vi "Mixed mode s-parameter conversion.vi"() -> ()   [LabVIEW 2020]
uses:
  <vilib>/Analysis/baseanly.llb/Complex A x B.vi
  <vilib>/addons/HF Network Analysis/Support VIs/Read SnP File (SnP).vi
  <vilib>/Analysis/Matrix/Numeric/Conversions/Array To Matrix - CA2.vi
  <vilib>/Analysis/Matrix/Numeric/Multiply/Multiply - CM,C.vi
  <vilib>/Analysis/baseanly.llb/Complex Inverse Matrix.vi
  <vilib>/Analysis/Matrix/Numeric/Conversions/Matrix To Array - CM.vi
  <vilib>/addons/HF Network Analysis/NI_HFNetworkAnalysis.lvlib
  <vilib>/Analysis/Matrix/NI_Matrix.lvlib
  <vilib>/Analysis/NI_AALBase.lvlib
panel:
  in  "Mixed mode port assignment":enum16{"a", "b"}(ring)
  in  "Direction":T1(ring)
  in  "SnP File Path":path
  # "Input file"
  # "Port assignment a (Keysight, R&S)\nSdd11 Sdc11 Sdd12 Sdc12\nScd11 Scc11  Scd12 Scc12\nSdd21 Sdc21 Sdd22 Sdc22\nScd21 Scc21 Scd22 Scc22\n\nPort assignment b (Dr. Bogatin, Dr. Dunsmore, ADS example)\nSdd11 Sdd12 Sdc11 Sdc12\nSdd21 Sdd22  Sdc21 Sdc22\nScd11 Scd12 Scc11 Scc12\nScd21 Scd22 Scc21 Scc22"
  # "Port assignment 4-port common mode\nS11 S12 S13 S14\nS21 S22 S23 S24\nS31 S32 S33 S34\nS41 S42 S43 S44"
  # "Single ended\nports"
  # "1\n\n3"
  # "2\n\n4"
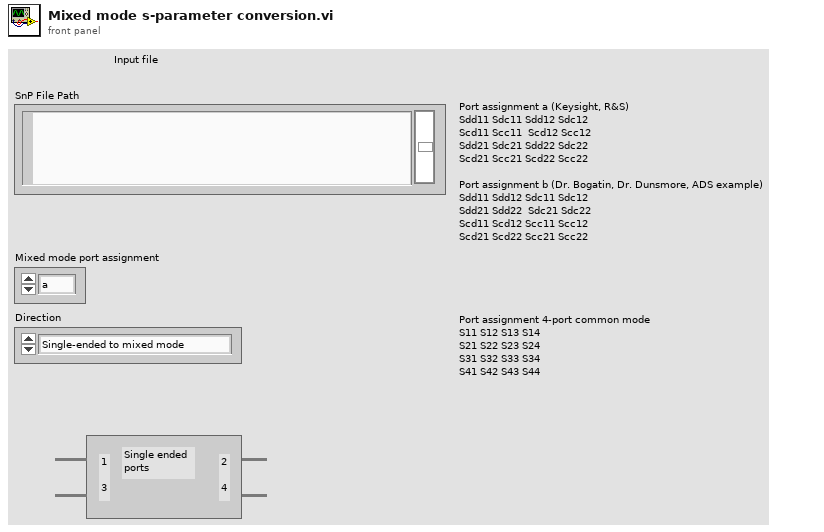
[diagram p1: front panel]
types:
  T1 = enum16{"Single-ended to mixed mode", "Mixed mode to single-ended"}
  T2 = typedef "NI_Matrix.lvlib/ComplexMatrix.ctl" = cdb[][]
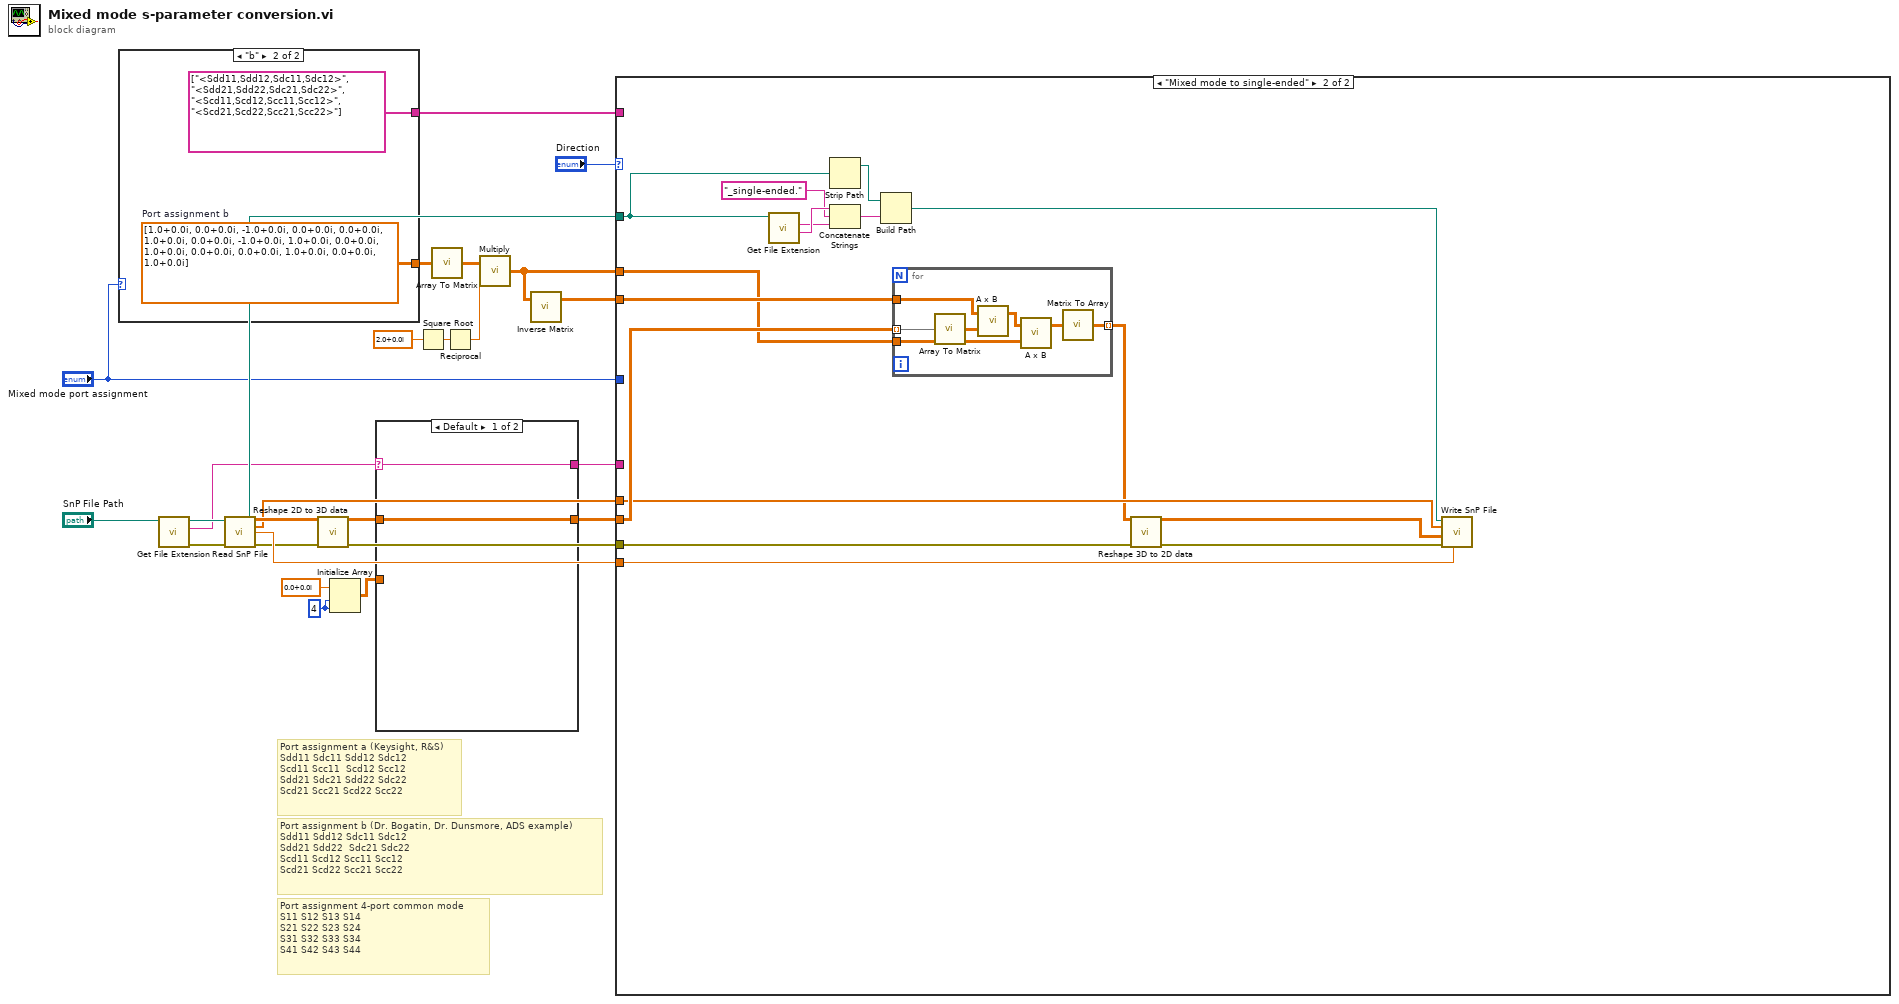
[diagram p0: block diagram]
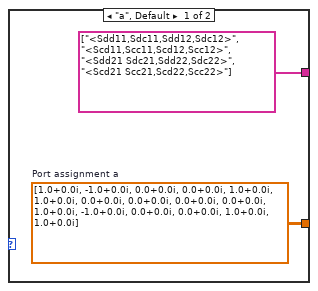
[diagram p2: hidden frame]
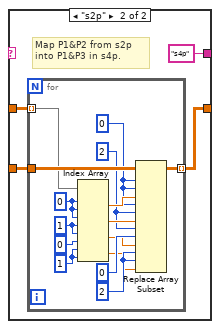
[diagram p3: hidden frame]
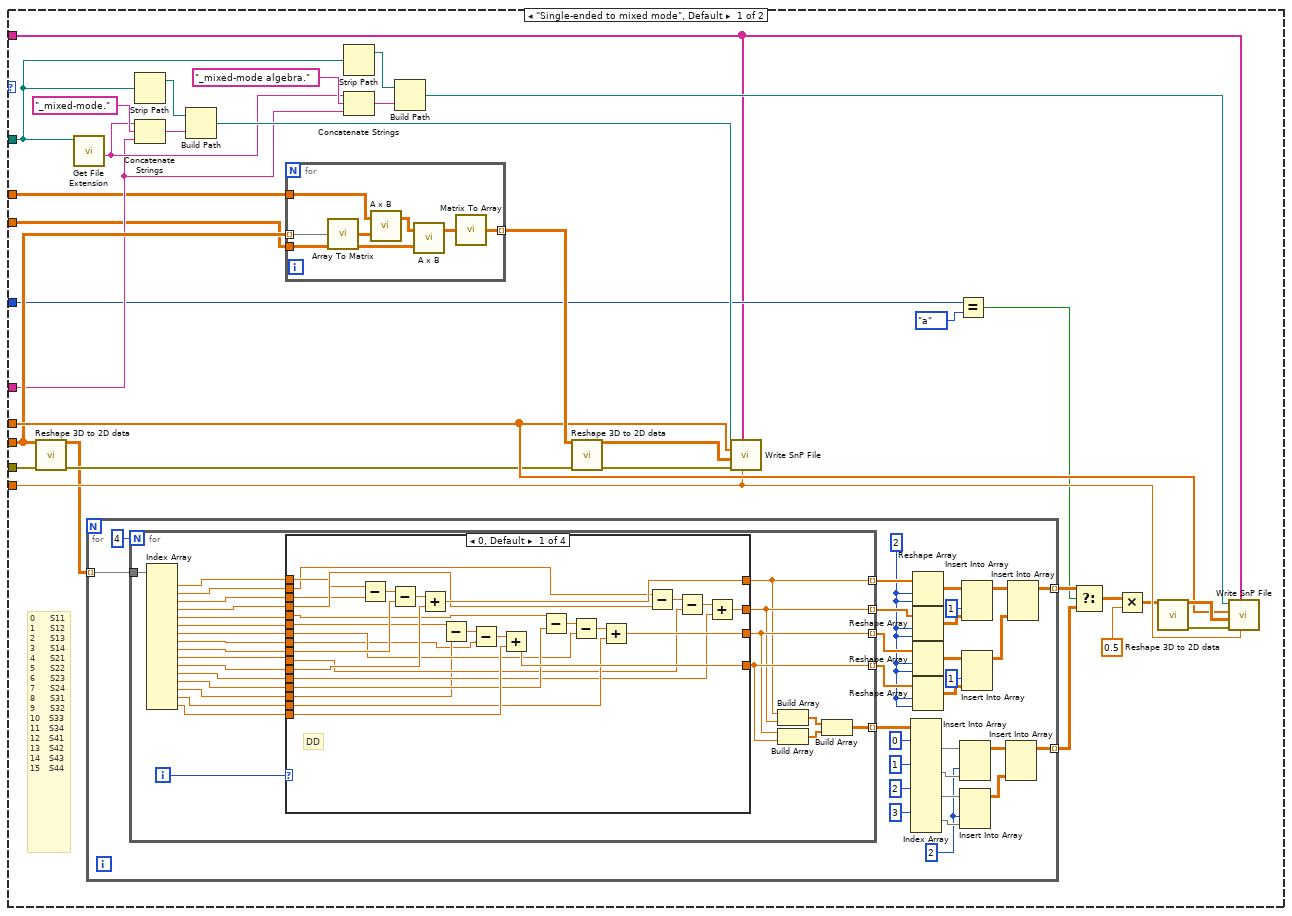
[diagram p4: hidden frame]
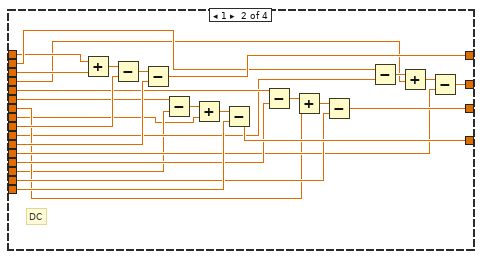
[diagram p5: hidden frame]
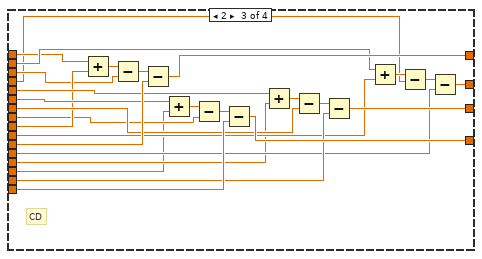
[diagram p6: hidden frame]
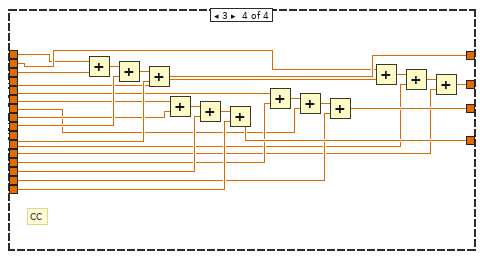
[diagram p7: hidden frame]
diagram:
  w3 = 4 ("dimension size")
  # "Port assignment 4-port common mode\nS11 S12 S13 S14\nS21 S22 S23 S24\nS31 S32 S33 S34\nS41 S42 S43 S44"
  # "Port assignment b (Dr. Bogatin, Dr. Dunsmore, ADS example)\nSdd11 Sdd12 Sdc11 Sdc12\nSdd21 Sdd22  Sdc21 Sdc22\nScd11 Scd12 Scc11 Scc12\nScd21 Scd22 Scc21 Scc22"
  # "Port assignment a (Keysight, R&S)\nSdd11 Sdc11 Sdd12 Sdc12\nScd11 Scc11  Scd12 Scc12\nSdd21 Sdc21 Sdd22 Sdc22\nScd21 Scc21 Scd22 Scc22"
  n1 = case shown="\"b\"" "Mixed mode port assignment" {
    tunnel: [w27 w29] -> w6
    tunnel: [string[] ["<Sdd11,Sdc11,Sdd12,Sdc12>", "<Scd11,Scc11,Scd12,Scc12>", "<Sdd21 Sdc21,Sdd22,Sdc22>", "<Scd21 Scc21,Scd22,Scc22>"] string[] ["<Sdd11,Sdd12,Sdc11,Sdc12>", "<Sdd21,Sdd22,Sdc21,Sdc22>", "<Scd11,Scd12,Scc11,Scc12>", "<Scd21,Scd22,Scc21,Scc22>"]] -> w1
    frame "a", Default {
      w27 = cdb[][] [[1.0+0.0i, -1.0+0.0i, 0.0+0.0i, 0.0+0.0i], [1.0+0.0i, 1.0+0.0i, 0.0+0.0i, 0.0+0.0i], [0.0+0.0i, 0.0+0.0i, 1.0+0.0i, -1.0+0.0i], [0.0+0.0i, 0.0+0.0i, 1.0+0.0i, 1.0+0.0i]]  # Port assignment a
    }
    frame "b" {
      w29 = cdb[][] [[1.0+0.0i, 0.0+0.0i, -1.0+0.0i, 0.0+0.0i], [0.0+0.0i, 1.0+0.0i, 0.0+0.0i, -1.0+0.0i], [1.0+0.0i, 0.0+0.0i, 1.0+0.0i, 0.0+0.0i], [0.0+0.0i, 1.0+0.0i, 0.0+0.0i, 1.0+0.0i]]  # Port assignment b
    }
  }
  n2 = call <vilib>:"Get File Extension.vi"("file"="SnP File Path") -> ("error out"=w17:errorcluster, "lowercase file extension"=w10:string, "dup file"=w18:path)  [unwired: 6 in, 2 out]
  n3 = call-poly <vilib>:"Read SnP File.vi"("SnP File Path"=w18, "Error In"=w17) -> ("S-parameters"=w16:cdb[][], "Frequencies (Hz)"=w13:dbl[], "Z0 (Ohm)"=w21:cdb, "Error Out"=w15:errorcluster)  [unwired: 10 in]
  n4 = call <vilib>:"Reshape 2D to 3D data.vi"("Parameters In (2D)"=w16, "Error In"=w15) -> ("Parameters Out (3D)"=w11:cdb[][][], "Error Out"=w14:errorcluster)  [unwired: 12 in]
  n5 = Initialize Array(cdb 0.0+0.0i, w3, w3) -> (w2:cdb[][])
  n6 = case shown="Default" w10 {
    selector: w10 -> [w30 _]
    tunnel: w2 -> [_ w34]
    tunnel: [w31 w35] -> w12
    tunnel: w11 -> [w31 w33]
    tunnel: [w30 "s4p" ("unmodified file extension")] -> w9
    frame Default {
    }
    frame "s2p" {
      # "Map P1&P2 from s2p\ninto P1&P3 in s4p."
      n7 = for {
        tunnel: w34 -> [w50]
        tunnel: w33 -> [w49] mode=indexing
        tunnel: [w36] -> w35 mode=indexing
        w38 = 2 ("index (col)")
        w41 = 2 ("disabled index (col)")
        w43 = 0 ("disabled index (col)")
        w45 = 1 ("index (col)")
        w47 = 1 ("disabled index (col)")
        w48 = 0 ("index (row)")
        n8 = Index Array(array=w49, index (row) #1=w48, index (col) #1=w48, index (row) #2=w48, index (col) #2=w47, index (row) #3=w47, index (col) #3=0 ("disabled index (col)"), index (row) #4=w45, index (col) #4=w45) -> (element #1=w44:cdb, element #2=w42:cdb, element #3=w39:cdb, element #4=w37:cdb)
        n9 = Replace Array Subset(array=w50, new element #1=w44, index (row) #1=w43, index (col) #1=w43, new element #2=w42, index (row) #2=w43, index (col) #2=w41, new element #3=w39, index (row) #3=w41, index (col) #3=0 ("disabled index (col)"), new element #4=w37, index (row) #4=w38, index (col) #4=w38) -> (w36:cdb[][])
      }
    }
  }
  n10 = Square Root(x=cdb 2.0+0.0i) -> (sqrt(x)=w24:cdb)
  n11 = call-poly <vilib>:"Array To Matrix.vi"("Complex 2D Array"=w6) -> ("Complex Matrix"=w23:T2)
  n12 = Reciprocal(x=w24) -> (1/x=w22:cdb)
  n13 = call-poly <vilib>:"Multiply.vi"("Complex Scalar c"=w22, "Complex Matrix A"=w23) -> ("A * c"=w8:T2)
  n14 = call-poly <vilib>:"Inverse Matrix.vi"("Input Matrix"=w8) -> ("Inverse Matrix"=w7:T2)  [unwired: 1 in, 1 out]
  n15 = case shown="\"Mixed mode to single-ended\"" "Direction" {
    tunnel: w12 -> [w62 w272]
    tunnel: w14 -> [w65 w271]
    tunnel: w13 -> [w69 w270]
    tunnel: w21 -> [w68 w269]
    tunnel: w18 -> [w71 w265]
    tunnel: w8 -> [w52 w257]
    tunnel: w9 -> [w61 _]
    tunnel: w7 -> [w51 w258]
    tunnel: "Mixed mode port assignment" -> [w54 _]
    tunnel: w1 -> [w53 _]
    frame "Single-ended to mixed mode", Default {
      # "0     S11\n1     S12\n2     S13\n3     S14\n4     S21\n5     S22\n6     S23\n7     S24\n8     S31\n9     S32\n10   S33\n11   S34\n12   S41\n13   S42\n14   S43\n15   S44"
      n16 = call <vilib>:"Reshape 3D to 2D data.vi"("Parameters In (3D)"=w62, "Error In"=w65) -> ("Parameters Out (2D)"=w63:cdb[][], "Error Out"=w64:errorcluster)  [unwired: 12 in]
      n17 = call <vilib>:"Get File Extension.vi"("file"=w71) -> ("filename without extension"=w72:string)  [unwired: 6 in, 4 out]
      n18 = for {
        tunnel: w63 -> [w112] mode=indexing
        tunnel: [w99] -> w60 mode=indexing
        tunnel: [w85] -> w59 mode=indexing
        w84 = 2 ("disabled index (col)")
        w106 = 2 ("dimension size")
        n19 = for {
          N: 4 -> [_]
          tunnel: w112 -> [w121]
          tunnel: [w116] -> w110 mode=indexing
          tunnel: [w117] -> w109 mode=indexing
          tunnel: [w118] -> w108 mode=indexing
          tunnel: [w119] -> w107 mode=indexing
          tunnel: [w135] -> w96 mode=indexing
          i -> [w120]
          n20 = Index Array(array=w121) -> (element #1=w134:cdb, element #2=w133:cdb, element #3=w132:cdb, element #4=w115:cdb, element #5=w114:cdb, element #6=w113:cdb, element #7=w131:cdb, element #8=w130:cdb, element #9=w129:cdb, element #10=w128:cdb, element #11=w127:cdb, element #12=w126:cdb, element #13=w125:cdb, element #14=w124:cdb, element #15=w123:cdb, element #16=w122:cdb)  [unwired: 16 in]
          n21 = case shown="0, Default" w120 {
            tunnel: [w157 w185 w213 w241] -> w116
            tunnel: [w156 w184 w212 w240] -> w119
            tunnel: [w155 w183 w211 w239] -> w118
            tunnel: [w154 w182 w210 w238] -> w117
            tunnel: w122 -> [w153 w181 w209 w237]
            tunnel: w123 -> [w152 w180 w208 w236]
            tunnel: w124 -> [w139 w167 w194 w235]
            tunnel: w125 -> [w151 w179 w196 w234]
            tunnel: w126 -> [w150 w178 w207 w233]
            tunnel: w127 -> [w149 w177 w206 w232]
            tunnel: w128 -> [w148 w168 w197 w231]
            tunnel: w129 -> [w147 w176 w200 w230]
            tunnel: w130 -> [w138 w166 w195 w229]
            tunnel: w131 -> [w146 w175 w205 w228]
            tunnel: w113 -> [w145 w174 w204 w227]
            tunnel: w114 -> [w144 w173 w203 w226]
            tunnel: w115 -> [w143 w169 w198 w225]
            tunnel: w132 -> [w142 w172 w199 w224]
            tunnel: w133 -> [w140 w171 w202 w223]
            tunnel: w134 -> [w141 w170 w201 w222]
            frame 0, Default {
              # "DD"
              n22 = Subtract(x=w141, y=w142) -> (x-y=w165:cdb)
              n23 = Subtract(x=w165, y=w147) -> (x-y=w164:cdb)
              n24 = Add(x=w164, y=w149) -> (x+y=w157:cdb)
              n25 = Subtract(x=w145, y=w139) -> (x-y=w162:cdb)
              n26 = Subtract(x=w162, y=w138) -> (x-y=w163:cdb)
              n27 = Add(x=w163, y=w153) -> (x+y=w156:cdb)
              n28 = Subtract(x=w144, y=w151) -> (x-y=w161:cdb)
              n29 = Subtract(x=w161, y=w146) -> (x-y=w160:cdb)
              n30 = Add(x=w160, y=w152) -> (x+y=w155:cdb)
              n31 = Subtract(x=w140, y=w143) -> (x-y=w159:cdb)
              n32 = Subtract(x=w159, y=w148) -> (x-y=w158:cdb)
              n33 = Add(x=w158, y=w150) -> (x+y=w154:cdb)
            }
            frame 1 {
              # "DC"
              n34 = Add(x=w170, y=w172) -> (x+y=w193:cdb)
              n35 = Subtract(x=w193, y=w176) -> (x-y=w192:cdb)
              n36 = Subtract(x=w192, y=w177) -> (x-y=w185:cdb)
              n37 = Subtract(x=w174, y=w167) -> (x-y=w190:cdb)
              n38 = Add(x=w190, y=w166) -> (x+y=w191:cdb)
              n39 = Subtract(x=w191, y=w181) -> (x-y=w184:cdb)
              n40 = Subtract(x=w173, y=w179) -> (x-y=w189:cdb)
              n41 = Add(x=w189, y=w175) -> (x+y=w188:cdb)
              n42 = Subtract(x=w188, y=w180) -> (x-y=w183:cdb)
              n43 = Subtract(x=w171, y=w168) -> (x-y=w187:cdb)
              n44 = Add(x=w187, y=w169) -> (x+y=w186:cdb)
              n45 = Subtract(x=w186, y=w178) -> (x-y=w182:cdb)
            }
            frame 2 {
              # "CD"
              n46 = Add(x=w201, y=w200) -> (x+y=w221:cdb)
              n47 = Subtract(x=w221, y=w199) -> (x-y=w220:cdb)
              n48 = Subtract(x=w220, y=w206) -> (x-y=w213:cdb)
              n49 = Add(x=w204, y=w194) -> (x+y=w218:cdb)
              n50 = Subtract(x=w218, y=w195) -> (x-y=w219:cdb)
              n51 = Subtract(x=w219, y=w209) -> (x-y=w212:cdb)
              n52 = Add(x=w203, y=w196) -> (x+y=w217:cdb)
              n53 = Subtract(x=w217, y=w205) -> (x-y=w216:cdb)
              n54 = Subtract(x=w216, y=w208) -> (x-y=w211:cdb)
              n55 = Add(x=w202, y=w197) -> (x+y=w215:cdb)
              n56 = Subtract(x=w215, y=w198) -> (x-y=w214:cdb)
              n57 = Subtract(x=w214, y=w207) -> (x-y=w210:cdb)
            }
            frame 3 {
              # "CC"
              n58 = Add(x=w222, y=w224) -> (x+y=w249:cdb)
              n59 = Add(x=w249, y=w230) -> (x+y=w248:cdb)
              n60 = Add(x=w248, y=w232) -> (x+y=w241:cdb)
              n61 = Add(x=w227, y=w229) -> (x+y=w246:cdb)
              n62 = Add(x=w246, y=w235) -> (x+y=w247:cdb)
              n63 = Add(x=w247, y=w237) -> (x+y=w240:cdb)
              n64 = Add(x=w226, y=w234) -> (x+y=w245:cdb)
              n65 = Add(x=w245, y=w228) -> (x+y=w244:cdb)
              n66 = Add(x=w244, y=w236) -> (x+y=w239:cdb)
              n67 = Add(x=w223, y=w225) -> (x+y=w243:cdb)
              n68 = Add(x=w243, y=w231) -> (x+y=w242:cdb)
              n69 = Add(x=w242, y=w233) -> (x+y=w238:cdb)
            }
          }
          n70 = Build Array(w116, w117) -> (w137:cdb[])
          n71 = Build Array(w118, w119) -> (w136:cdb[])
          n72 = Build Array(w137, w136) -> (w135:cdb[][])
        }
        n73 = Index Array(array=w96, index (dim 0) #1=0 ("index (page)"), index (dim 0) #2=1 ("index (page)"), index (dim 0) #3=2 ("index (page)"), index (dim 0) #4=3 ("index (page)")) -> (element #1=w91:cdb[][], element #2=w90:cdb[][], element #3=w89:cdb[][], element #4=w88:cdb[][])  [unwired: 8 in]
        n74 = Reshape Array(w110, w106, w106) -> (w105:cdb[][])
        n75 = Reshape Array(w109, w106, w106) -> (w104:cdb[][])
        n76 = Reshape Array(w108, w106, w106) -> (w103:cdb[][])
        n77 = Reshape Array(w107, w106, w106) -> (w102:cdb[][])
        n78 = Insert Into Array(array=w91, index (col)=w84, new element=w90) -> (w86:cdb[][])  [unwired: 1 in]
        n79 = Insert Into Array(array=w89, index (col)=w84, new element=w88) -> (w87:cdb[][])  [unwired: 1 in]
        n80 = Insert Into Array(array=w105, index (col)=1 ("disabled index (col)"), new element=w104) -> (w101:cdb[][])  [unwired: 1 in]
        n81 = Insert Into Array(array=w103, index (col)=1 ("disabled index (col)"), new element=w102) -> (w100:cdb[][])  [unwired: 1 in]
        n82 = Insert Into Array(array=w86, new element=w87) -> (w85:cdb[][])  [unwired: 2 in]
        n83 = Insert Into Array(array=w101, new element=w100) -> (w99:cdb[][])  [unwired: 2 in]
      }
      n84 = Strip Path(path=w71) -> (stripped path=w80:path)  [unwired: 1 out]
      n85 = Concatenate Strings(w72, "_mixed-mode." ("string"), w61) -> (w81:string)
      n86 = Build Path(base path=w80, name or relative path=w81) -> (appended path=w79:path)
      n87 = for {
        tunnel: w62 -> [w256] mode=indexing
        tunnel: w52 -> [w254]
        tunnel: w51 -> [w252]
        tunnel: [w255] -> w78 mode=indexing
        n88 = call-poly <vilib>:"Array To Matrix.vi"("Complex 2D Array"=w256) -> ("Complex Matrix"=w253:T2)
        n89 = call-poly <vilib>:"A x B.vi"("B"=w253, "A"=w254) -> ("A x B"=w251:T2)  [unwired: 1 out]
        n90 = call-poly <vilib>:"A x B.vi"("B"=w252, "A"=w251) -> ("A x B"=w250:T2)  [unwired: 1 out]
        n91 = call-poly <vilib>:"Matrix To Array.vi"("Complex Matrix"=w250) -> ("Complex 2D Array"=w255:cdb[][])
      }
      n92 = Strip Path(path=w71) -> (stripped path=w75:path)  [unwired: 1 out]
      n93 = Concatenate Strings(w72, "_mixed-mode algebra." ("string"), w61) -> (w74:string)
      n94 = Build Path(base path=w75, name or relative path=w74) -> (appended path=w70:path)
      n95 = call <vilib>:"Reshape 3D to 2D data.vi"("Parameters In (3D)"=w78, "Error In"=w64) -> ("Parameters Out (2D)"=w55:cdb[][], "Error Out"=w83:errorcluster)  [unwired: 12 in]
      n96 = call <vilib>:"Write SnP File.vi"("Z0 (50 Ohm)"=w68, "Comments"=w53, "error in (no error)"=w83, "S-parameters"=w55, "Frequencies (Hz)"=w69, "SnP File Path"=w79) -> ()  [unwired: 5 in, 1 out]
      n97 = Equal?(x=w54, y=enum16{"a", "b"}."a") -> (x = y?=w57:bool)
      n98 = Select(t=w60, s=w57, f=w59) -> (s? t:f=w56:cdb[][][])
      n99 = Multiply(x=w56, y=0.5) -> (x*y=w67:cdb[][][])
      n100 = call <vilib>:"Reshape 3D to 2D data.vi"("Parameters In (3D)"=w67) -> ("Parameters Out (2D)"=w77:cdb[][], "Error Out"=w76:errorcluster)  [unwired: 13 in]
      n101 = call <vilib>:"Write SnP File.vi"("Z0 (50 Ohm)"=w68, "Comments"=w53, "error in (no error)"=w76, "S-parameters"=w77, "Frequencies (Hz)"=w69, "SnP File Path"=w70) -> ()  [unwired: 5 in, 1 out]
    }
    frame "Mixed mode to single-ended" {
      n102 = call <vilib>:"Get File Extension.vi"("file"=w265) -> ("filename without extension"=w267:string, "lowercase file extension"=w264:string)  [unwired: 6 in, 3 out]
      n103 = Strip Path(path=w265) -> (stripped path=w262:path)  [unwired: 1 out]
      n104 = Concatenate Strings(w267, "_single-ended." ("string"), w264) -> (w263:string)
      n105 = Build Path(base path=w262, name or relative path=w263) -> (appended path=w261:path)
      n106 = for {
        tunnel: w272 -> [w279] mode=indexing
        tunnel: w258 -> [w277]
        tunnel: w257 -> [w275]
        tunnel: [w278] -> w260 mode=indexing
        n107 = call-poly <vilib>:"Array To Matrix.vi"("Complex 2D Array"=w279) -> ("Complex Matrix"=w276:T2)
        n108 = call-poly <vilib>:"A x B.vi"("B"=w276, "A"=w277) -> ("A x B"=w274:T2)  [unwired: 1 out]
        n109 = call-poly <vilib>:"A x B.vi"("B"=w275, "A"=w274) -> ("A x B"=w273:T2)  [unwired: 1 out]
        n110 = call-poly <vilib>:"Matrix To Array.vi"("Complex Matrix"=w273) -> ("Complex 2D Array"=w278:cdb[][])
      }
      n111 = call <vilib>:"Reshape 3D to 2D data.vi"("Parameters In (3D)"=w260, "Error In"=w271) -> ("Parameters Out (2D)"=w259:cdb[][], "Error Out"=w268:errorcluster)  [unwired: 12 in]
      n112 = call <vilib>:"Write SnP File.vi"("Z0 (50 Ohm)"=w269, "error in (no error)"=w268, "S-parameters"=w259, "Frequencies (Hz)"=w270, "SnP File Path"=w261) -> ()  [unwired: 6 in, 1 out]
    }
  }
